vi "Global_OnCommand.vi"(10 "Command ID":string, 11 "Object":T1) -> ()   [LabVIEW 2020, in "Project Provider.lvlib"]
uses:
  Project Provider.lvlib
  <resource>/Framework/Providers/API/ItemRef.ctl
panel:
  out "error out":errorcluster
  in  "error in":errorcluster
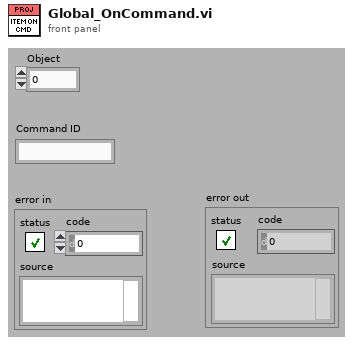
[diagram p1: front panel]
types:
  T1 = typedef "ItemRef.ctl" = u64
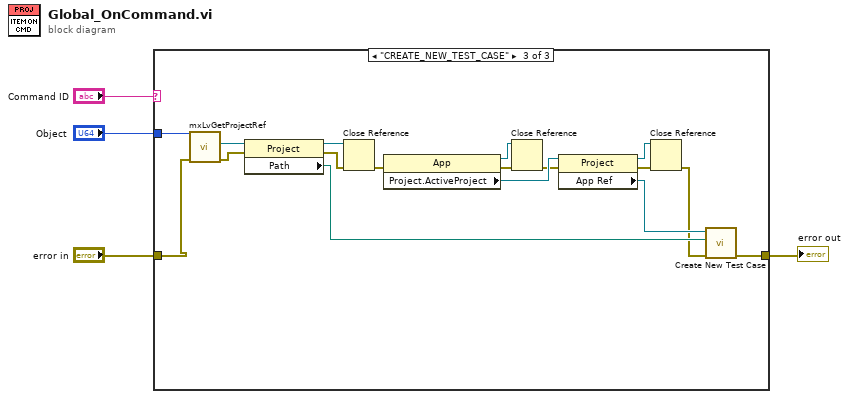
[diagram p0: block diagram]
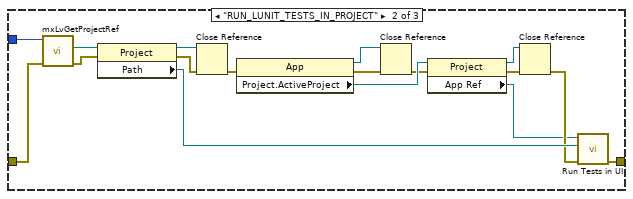
[diagram p3: hidden frame]
diagram:
  n1 = case shown="\"CREATE_NEW_TEST_CASE\"" "Command ID" {
    tunnel: "error in" -> [w5 w17 w26]
    tunnel: [w5 w20 w39] -> w2
    tunnel: "Object" -> [_ w18 w27]
    frame Default {
    }
    frame "RUN_LUNIT_TESTS_IN_PROJECT" {
      n2 = call <resource>:"mxLvGetProjectRef.vi"("error in"=w17, "Item"=w18) -> ("error out"=w15:errorcluster, "Project Refnum"=w16:refnum<vi>)  [unwired: 7 in, 1 out]
      n3 = property class="Project"(reference=w16, error in=w15) -> (reference out=w21:refnum<vi>, error out=w22:errorcluster, "Path"=w19:path)
      n4 = Close Reference(reference=w21, error in (no error)=w22) -> (error out=w8:errorcluster)
      n5 = property class="App"(error in=w8) -> (reference out=w9:refnum<vi>, error out=w11:errorcluster, "Project.ActiveProject"=w14:refnum<vi>)  [unwired: 1 in]
      n6 = Close Reference(reference=w9, error in (no error)=w11) -> (error out=w10:errorcluster)
      n7 = property class="Project"(reference=w14, error in=w10) -> (reference out=w13:refnum<vi>, error out=w12:errorcluster, "App Ref"=w6:refnum<vi>)
      n8 = Close Reference(reference=w13, error in (no error)=w12) -> (error out=w7:errorcluster)
      n9 = call "Run Tests in UI.vi"("error in (no error)"=w7, "Path"=w19, "Application"=w6) -> ("error out"=w20:errorcluster)  [unwired: 8 in]
    }
    frame "CREATE_NEW_TEST_CASE" {
      n10 = call <resource>:"mxLvGetProjectRef.vi"("error in"=w26, "Item"=w27) -> ("error out"=w35:errorcluster, "Project Refnum"=w36:refnum<vi>)  [unwired: 7 in, 1 out]
      n11 = property class="Project"(reference=w36, error in=w35) -> (reference out=w37:refnum<vi>, error out=w38:errorcluster, "Path"=w25:path)
      n12 = Close Reference(reference=w37, error in (no error)=w38) -> (error out=w28:errorcluster)
      n13 = property class="App"(error in=w28) -> (reference out=w29:refnum<vi>, error out=w31:errorcluster, "Project.ActiveProject"=w34:refnum<vi>)  [unwired: 1 in]
      n14 = Close Reference(reference=w29, error in (no error)=w31) -> (error out=w30:errorcluster)
      n15 = property class="Project"(reference=w34, error in=w30) -> (reference out=w33:refnum<vi>, error out=w32:errorcluster, "App Ref"=w24:refnum<vi>)
      n16 = Close Reference(reference=w33, error in (no error)=w32) -> (error out=w23:errorcluster)
      n17 = call "Create New Test Case.vi"("error in (no error)"=w23, "Path"=w25, "Application"=w24) -> ("error out"=w39:errorcluster)  [unwired: 8 in]
    }
  }
  "error out" <- w2
